vi "Unescape JSON string.vi"(8 "error in (no error)":errorcluster, 11 "Text (with JSON escapes)":string) -> (0 "error out":errorcluster, 3 "Text (unescaped)":string)   [LabVIEW 2020, in "JSONtext.lvlib"]
uses:
  <vilib>/JDP Science/JSONtext/JSONtext.lvlib
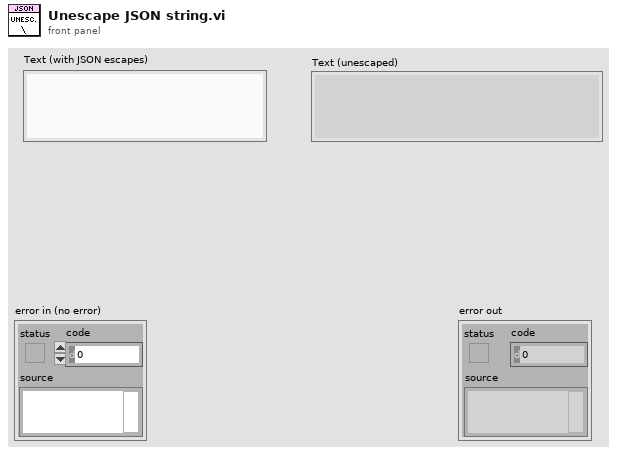
[diagram p1: front panel]
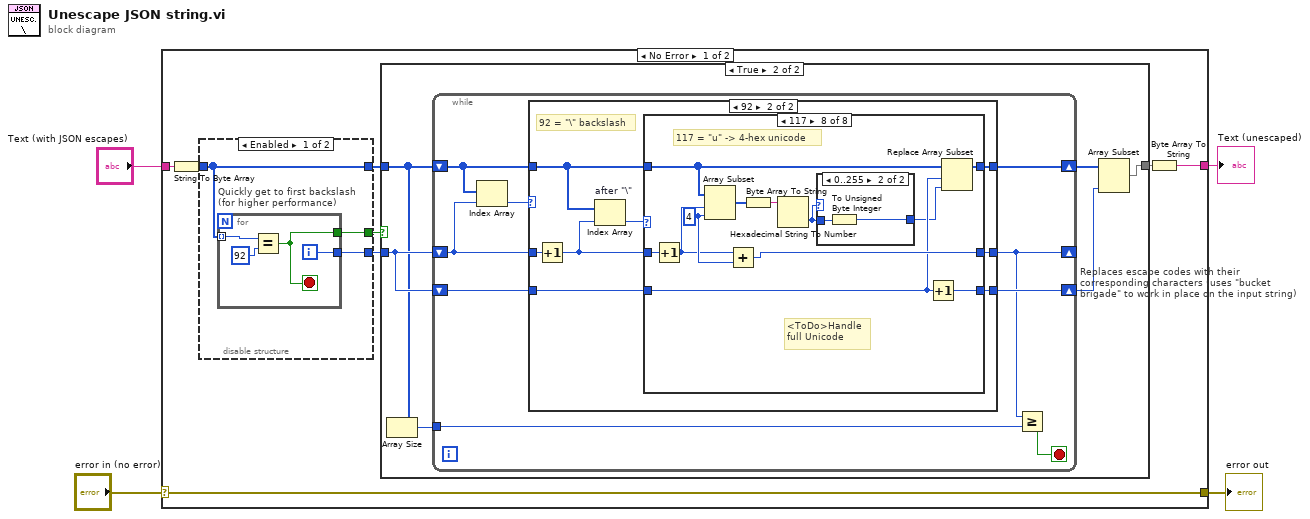
[diagram p0: block diagram]
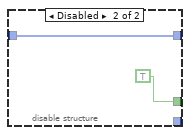
[diagram p2: hidden frame]
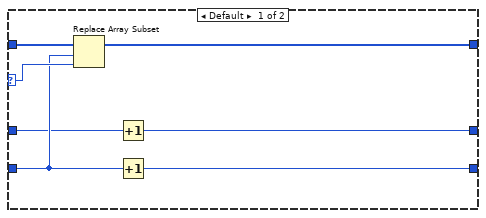
[diagram p4: hidden frame]
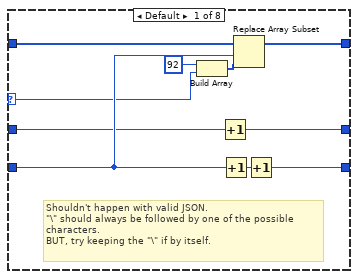
[diagram p5: hidden frame]
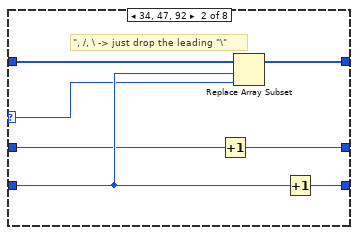
[diagram p6: hidden frame]
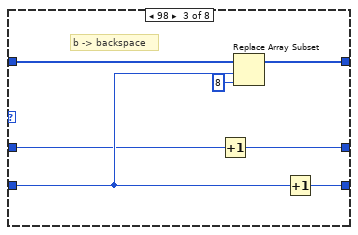
[diagram p7: hidden frame]
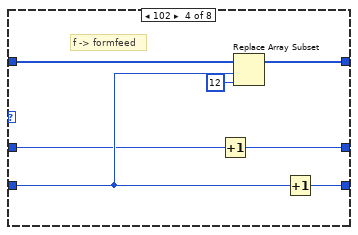
[diagram p8: hidden frame]
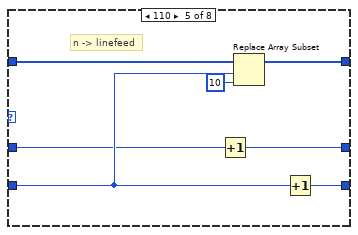
[diagram p9: hidden frame]
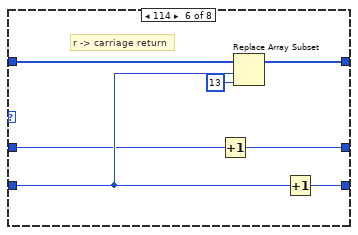
[diagram p10: hidden frame]
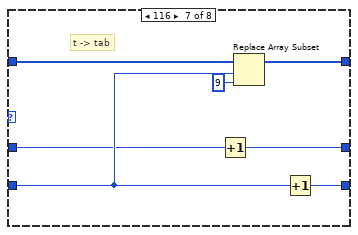
[diagram p11: hidden frame]
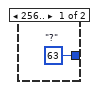
[diagram p12: hidden frame]
diagram:
  n1 = case shown="No Error" "error in (no error)" {
    selector: "error in (no error)" -> [w12 w121]
    tunnel: [w12 w121] -> w3
    tunnel: "Text (with JSON escapes)" -> [w11 w120]
    tunnel: [w9 w120] -> w1
    frame No Error {
      n2 = String To Byte Array(string=w11) -> (unsigned byte array=w8:u8[])
      n3 = disable-structure shown="Enabled" {
        disable-tunnel: w8 -> [w13 w21]
        disable-tunnel: [w15 _] -> w7
        disable-tunnel: [w13 w21] -> w6
        disable-tunnel: [w14 TRUE] -> w5
        frame Enabled {
          n4 = for "Quickly get to first backslash\n(for higher performance)" {
            tunnel: w13 -> [w18] mode=indexing
            tunnel: [w17] -> w15
            tunnel: [w16] -> w14
            i -> [w17]
            stop <- w16 stop-if-true
            n5 = Equal?(x=w18, y=u8 92 ("new element/subarray")) -> (x = y?=w16:bool)
          }
        }
        frame Disabled {
        }
      }
      n6 = case shown="True" w5 {
        tunnel: [w22 w26] -> w10
        tunnel: w7 -> [_ w24]
        tunnel: w6 -> [w22 w23]
        frame False {
          # "No escapes in string"
        }
        frame True {
          n7 = Array Size(array=w23) -> (size(s)=w25:i32)
          n8 = while "Replaces escape codes with their corresponding characters (uses \"bucket brigade\" to work in place on the input string)" {
            shift-right: [w33] -> w28
            shift-left: w23 -> [w36]
            shift-right: [w30] -> _
            shift-left: w24 -> [w35]
            shift-right: [w32] -> w27
            shift-left: w24 -> [w34]
            tunnel: w25 -> [w29]
            stop <- w31 stop-if-true
            n9 = Index Array(array=w36, index=w35) -> (element=w37:u8)
            n10 = case shown="92" w37 {
              selector: w37 -> [w43 _]
              tunnel: w36 -> [w44 w50]
              tunnel: w35 -> [w40 w51]
              tunnel: w34 -> [w41 w47]
              tunnel: [w42 w48] -> w33
              tunnel: [w39 w45] -> w32
              tunnel: [w38 w46] -> w30
              frame Default {
                n11 = Replace Array Subset(array=w44, new element=w43, index=w41) -> (w42:u8[])
                n12 = Increment(x=w40) -> (x+1=w38:i32)
                n13 = Increment(x=w41) -> (x+1=w39:i32)
              }
              frame 92 {
                # "92 = \"\\\" backslash"
                n14 = Increment(x=w51) -> (x+1=w49:i32)
                n15 = Index Array "after \"\\\""(array=w50, index=w49) -> (element=w52:u8)
                n16 = case shown="117" w52 {
                  selector: w52 -> [w54 w63 _ _ _ _ _ _]
                  tunnel: w50 -> [w62 w69 w76 w83 w90 w97 w104 w114]
                  tunnel: w49 -> [w57 w65 w72 w79 w86 w93 w100 w112]
                  tunnel: [w61 w68 w75 w82 w89 w96 w103 w113] -> w48
                  tunnel: w47 -> [w58 w66 w73 w80 w87 w94 w101 w109]
                  tunnel: [w56 w64 w71 w78 w85 w92 w99 w110] -> w46
                  tunnel: [w53 w67 w74 w81 w88 w95 w102 w108] -> w45
                  frame Default {
                    # "Shouldn't happen with valid JSON.  \n\"\\\" should always be followed by one of the possible\ncharacters.\nBUT, try keeping the \"\\\" if by itself."
                    n17 = Build Array(u8 92 ("new element/subarray"), w54) -> (w55:u8[])
                    n18 = Increment(x=w57) -> (x+1=w56:i32)
                    n19 = Increment(x=w58) -> (x+1=w59:i32)
                    n20 = Replace Array Subset(array=w62, new element=w55, index=w58) -> (w61:u8[])
                    n21 = Increment(x=w59) -> (x+1=w53:i32)
                  }
                  frame 34, 47, 92 {
                    # "\", /, \\ -> just drop the leading \"\\\""
                    n22 = Increment(x=w65) -> (x+1=w64:i32)
                    n23 = Replace Array Subset(array=w69, new element=w63, index=w66) -> (w68:u8[])
                    n24 = Increment(x=w66) -> (x+1=w67:i32)
                  }
                  frame 98 {
                    # "b -> backspace"
                    n25 = Increment(x=w72) -> (x+1=w71:i32)
                    n26 = Replace Array Subset(array=w76, new element=u8 8 ("new element/subarray"), index=w73) -> (w75:u8[])
                    n27 = Increment(x=w73) -> (x+1=w74:i32)
                  }
                  frame 102 {
                    # "f -> formfeed"
                    n28 = Increment(x=w79) -> (x+1=w78:i32)
                    n29 = Replace Array Subset(array=w83, new element=u8 12 ("new element/subarray"), index=w80) -> (w82:u8[])
                    n30 = Increment(x=w80) -> (x+1=w81:i32)
                  }
                  frame 110 {
                    # "n -> linefeed"
                    n31 = Increment(x=w86) -> (x+1=w85:i32)
                    n32 = Replace Array Subset(array=w90, new element=u8 10 ("new element/subarray"), index=w87) -> (w89:u8[])
                    n33 = Increment(x=w87) -> (x+1=w88:i32)
                  }
                  frame 114 {
                    # "r -> carriage return"
                    n34 = Increment(x=w93) -> (x+1=w92:i32)
                    n35 = Replace Array Subset(array=w97, new element=u8 13 ("new element/subarray"), index=w94) -> (w96:u8[])
                    n36 = Increment(x=w94) -> (x+1=w95:i32)
                  }
                  frame 116 {
                    # "t -> tab"
                    n37 = Increment(x=w100) -> (x+1=w99:i32)
                    n38 = Replace Array Subset(array=w104, new element=u8 9 ("new element/subarray"), index=w101) -> (w103:u8[])
                    n39 = Increment(x=w101) -> (x+1=w102:i32)
                  }
                  frame 117 {
                    w111 = 4 ("length")
                    # "<ToDo>Handle\nfull Unicode"
                    # "117 = \"u\" -> 4-hex unicode"
                    n40 = Increment(x=w112) -> (x+1=w106:i32)
                    n41 = Array Subset(array=w114, index=w106, length=w111) -> (w116:u8[])
                    n42 = Add(x=w106, y=w111) -> (x+y=w110:i32)
                    n43 = Byte Array To String(unsigned byte array=w116) -> (string=w115:string)
                    n44 = Hexadecimal String To Number(string=w115) -> (number=w105:u32)  [unwired: 2 in, 1 out]
                    n45 = case shown="0..255" w105 {
                      tunnel: w105 -> [_ w119]
                      tunnel: [w117 w118] -> w107
                      frame 256.. {
                        w117 = u8 63  # "?"
                      }
                      frame 0..255 {
                        n46 = To Unsigned Byte Integer(number=w119) -> (unsigned 8bit integer=w118:u8)
                      }
                    }
                    n47 = Increment(x=w109) -> (x+1=w108:i32)
                    n48 = Replace Array Subset(array=w114, new element=w107, index=w109) -> (w113:u8[])
                  }
                }
              }
            }
            n49 = Greater Or Equal?(x=w30, y=w29) -> (x >= y?=w31:bool)
          }
          n50 = Array Subset(array=w28, length=w27) -> (w26:u8[])  [unwired: 1 in]
        }
      }
      n51 = Byte Array To String(unsigned byte array=w10) -> (string=w9:string)
    }
    frame Error {
    }
  }
  "error out" <- w3
  "Text (unescaped)" <- w1
